vi "random number.vi"() -> ()   [LabVIEW 2012]
panel:
  out "Numeric":i32
  in  "stop":bool
  out "Waveform Chart":dbl(graph)
  out "Thermometer":dbl(slide) scale=0.0..100.0
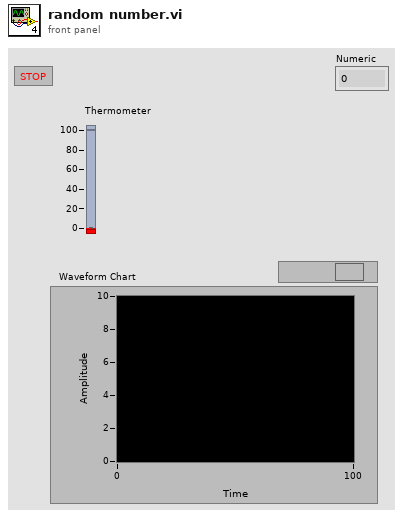
[diagram p1: front panel]
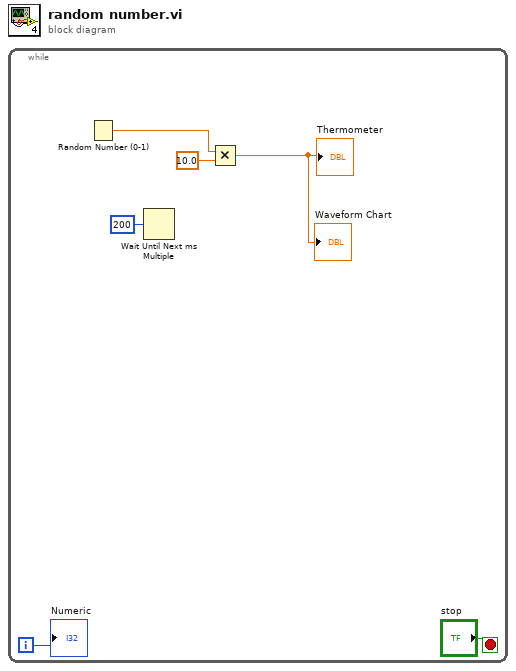
[diagram p0: block diagram]
diagram:
  n1 = while {
    i -> [w1]
    stop <- "stop" stop-if-true
    n2 = Random Number (0-1)() -> (number: 0 to 1=w4:dbl)
    n3 = Wait Until Next ms Multiple(millisecond multiple=u32 200) -> ()  [unwired: 1 out]
    n4 = Multiply(x=w4, y=10.0) -> (x*y=→"Thermometer" →"Waveform Chart":dbl)
    "Numeric" <- w1
  }
